vi "resonant.raw queue to image queue_MD.vi"() -> ()   [LabVIEW 2012]
uses:
  <vilib>/Utility/VariantDataType/Type.ctl
  GFG/GFGnumericGet.vi
  GFG/GFGbooleanGet.vi
  GFG/GFG library.lvlib
  <vilib>/Utility/VariantDataType/VariantType.lvlib
panel:
  out "size(s) 4":i32[](array[numeric])
  out "# elements in raw queue 2":i32
  out "error out 2":errorcluster
  out "error out 5":errorcluster
  out "size(s) 3":i32[](array[numeric])
  out "size(s) 2":i32[](array[numeric])
  out "size(s)":i32[](array[numeric])
  out "Numeric Control 2":i32
  out "Numeric Control":i32
  out "error out 4":errorcluster
  out "# elements in raw queue":i32
  out "error out":errorcluster
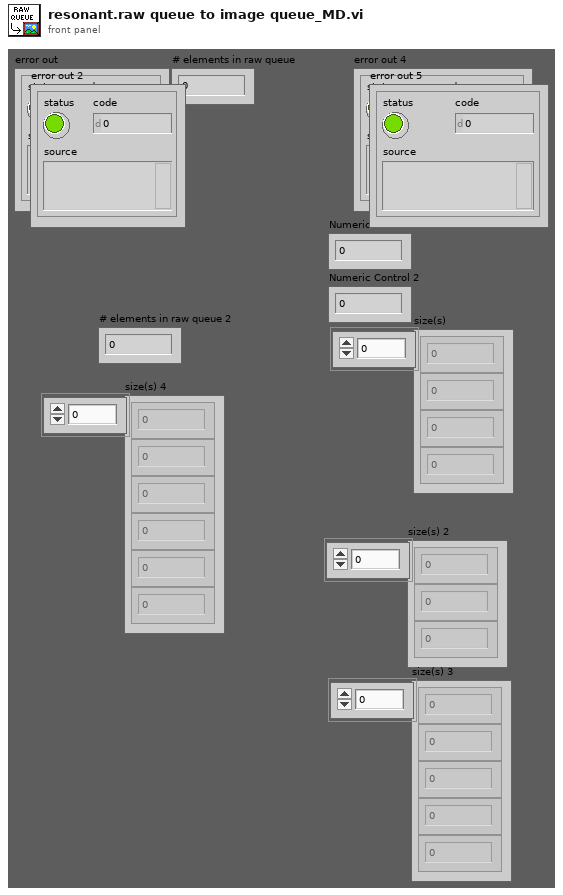
[diagram p1: front panel]
types:
  T1 = cluster{"NewVal":bool, "Event Registration Refnum":refnum<event-registration>}
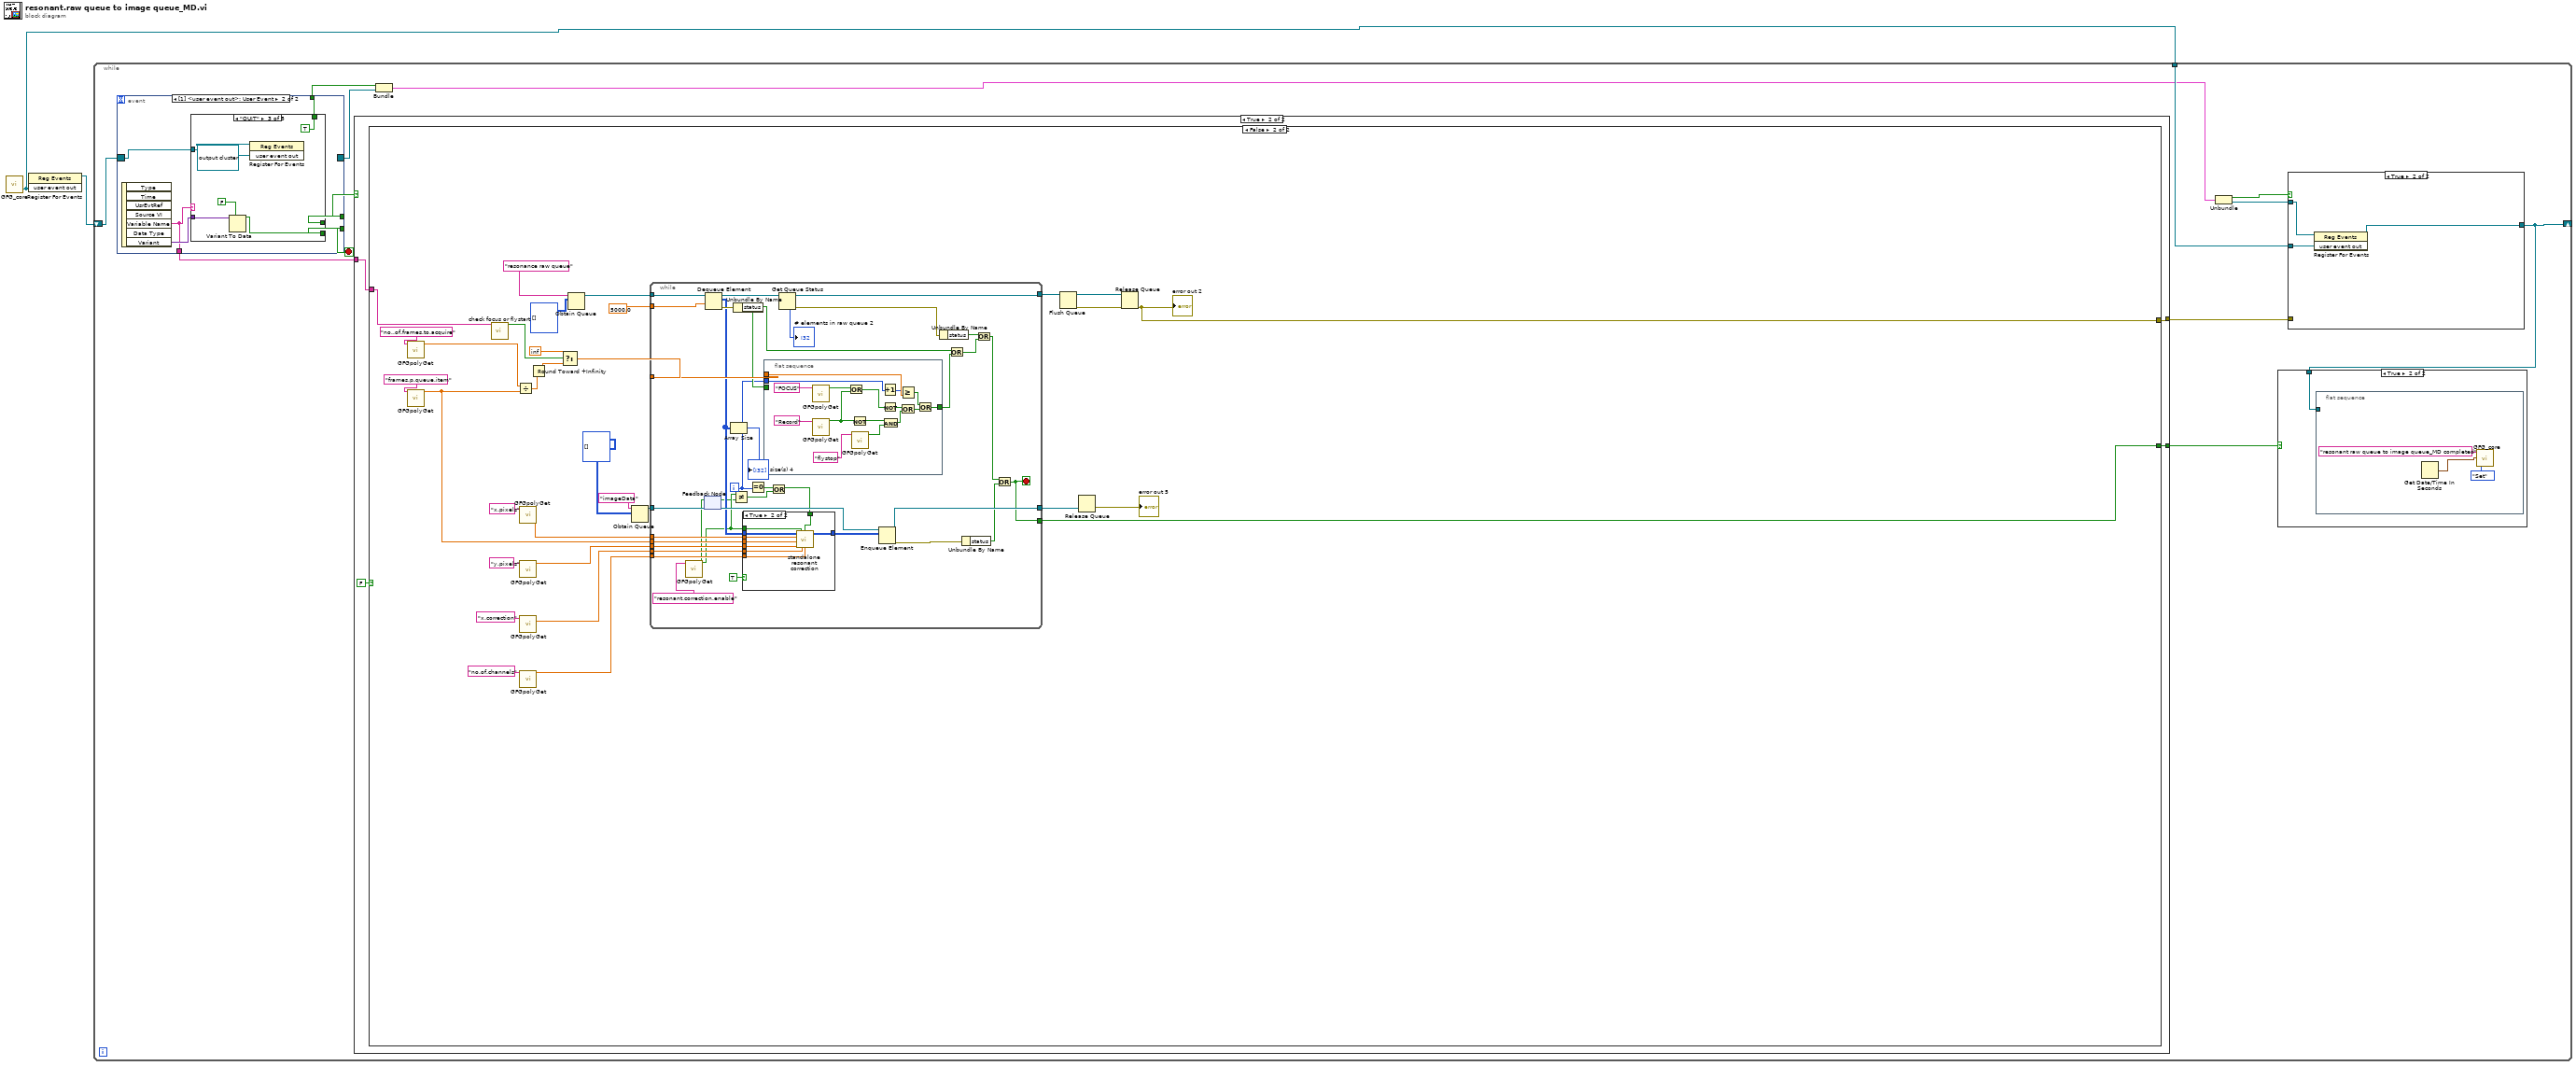
[diagram p0: block diagram]
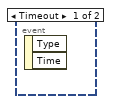
[diagram p4: hidden frame]
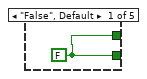
[diagram p5: hidden frame]
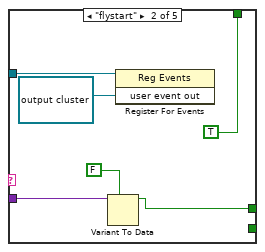
[diagram p6: hidden frame]
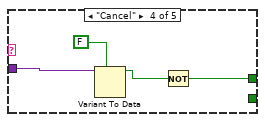
[diagram p7: hidden frame]
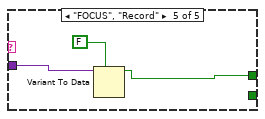
[diagram p8: hidden frame]
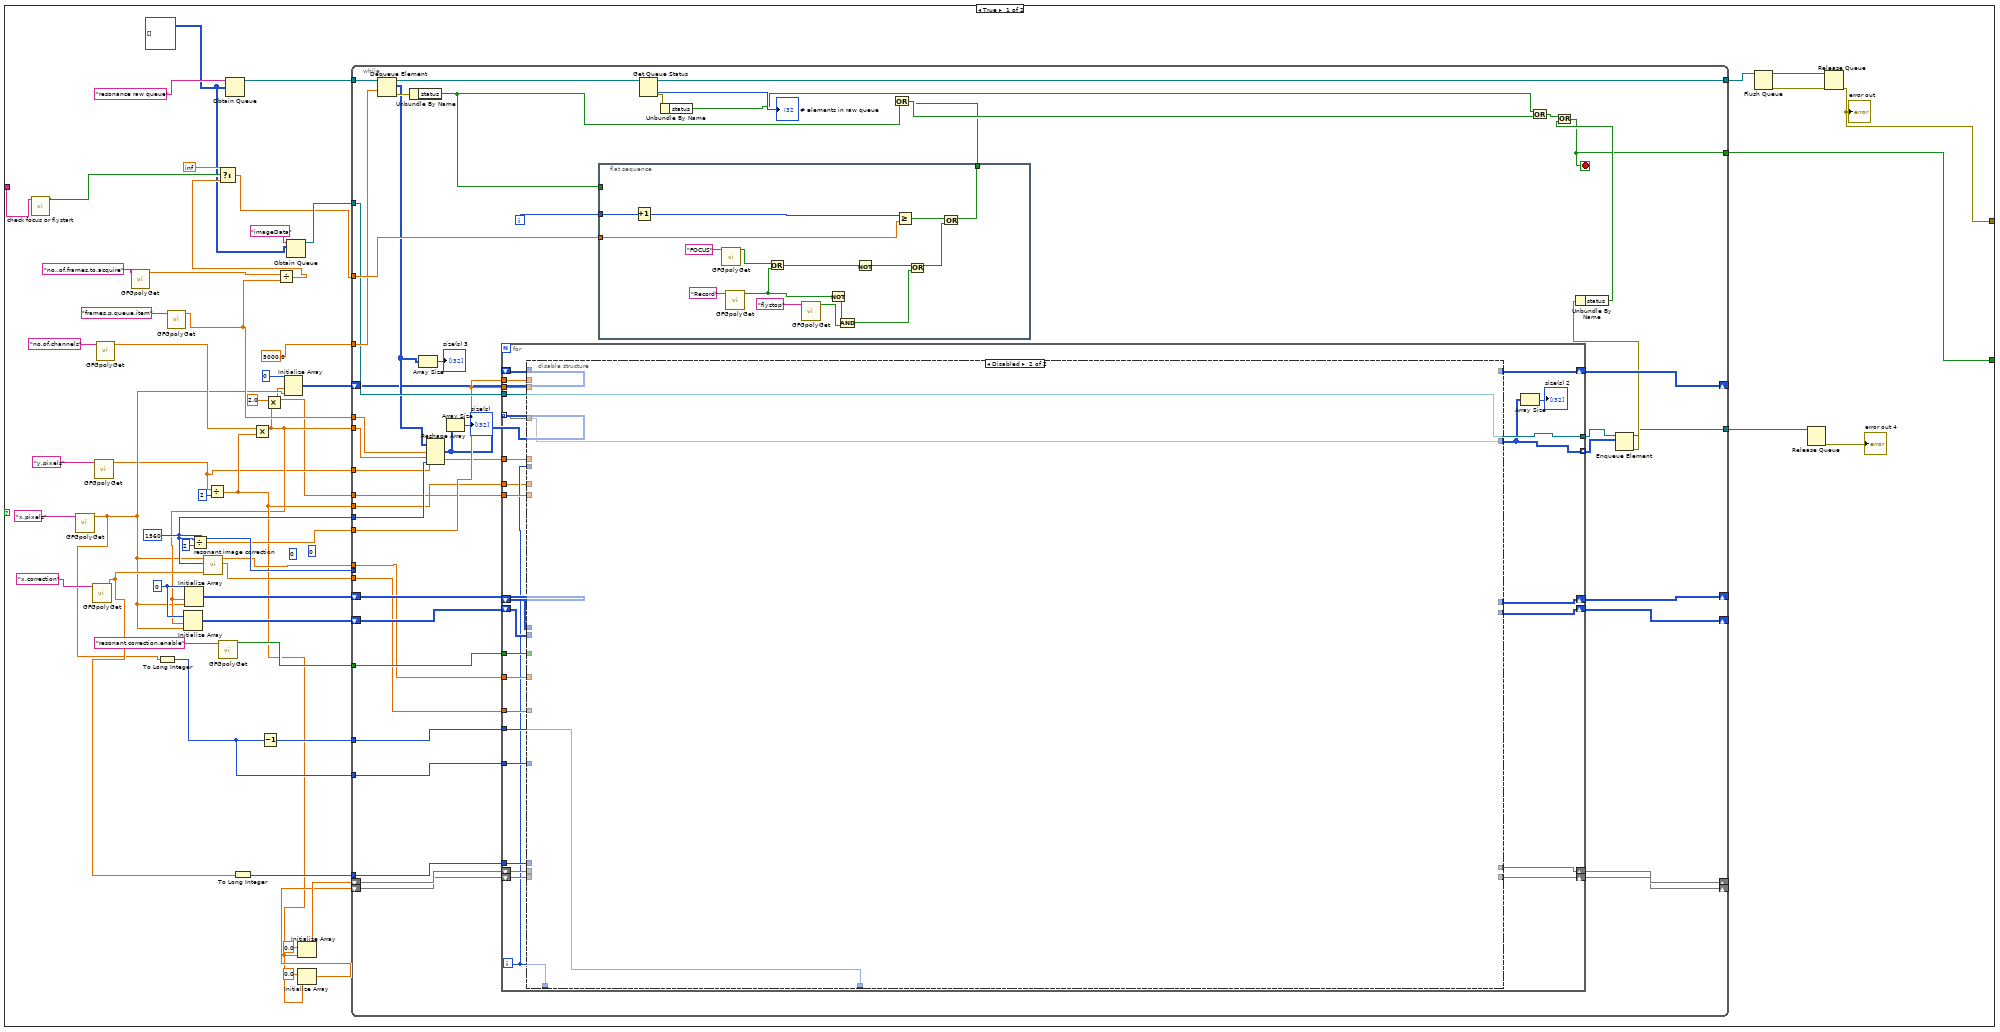
[diagram p10: hidden frame]
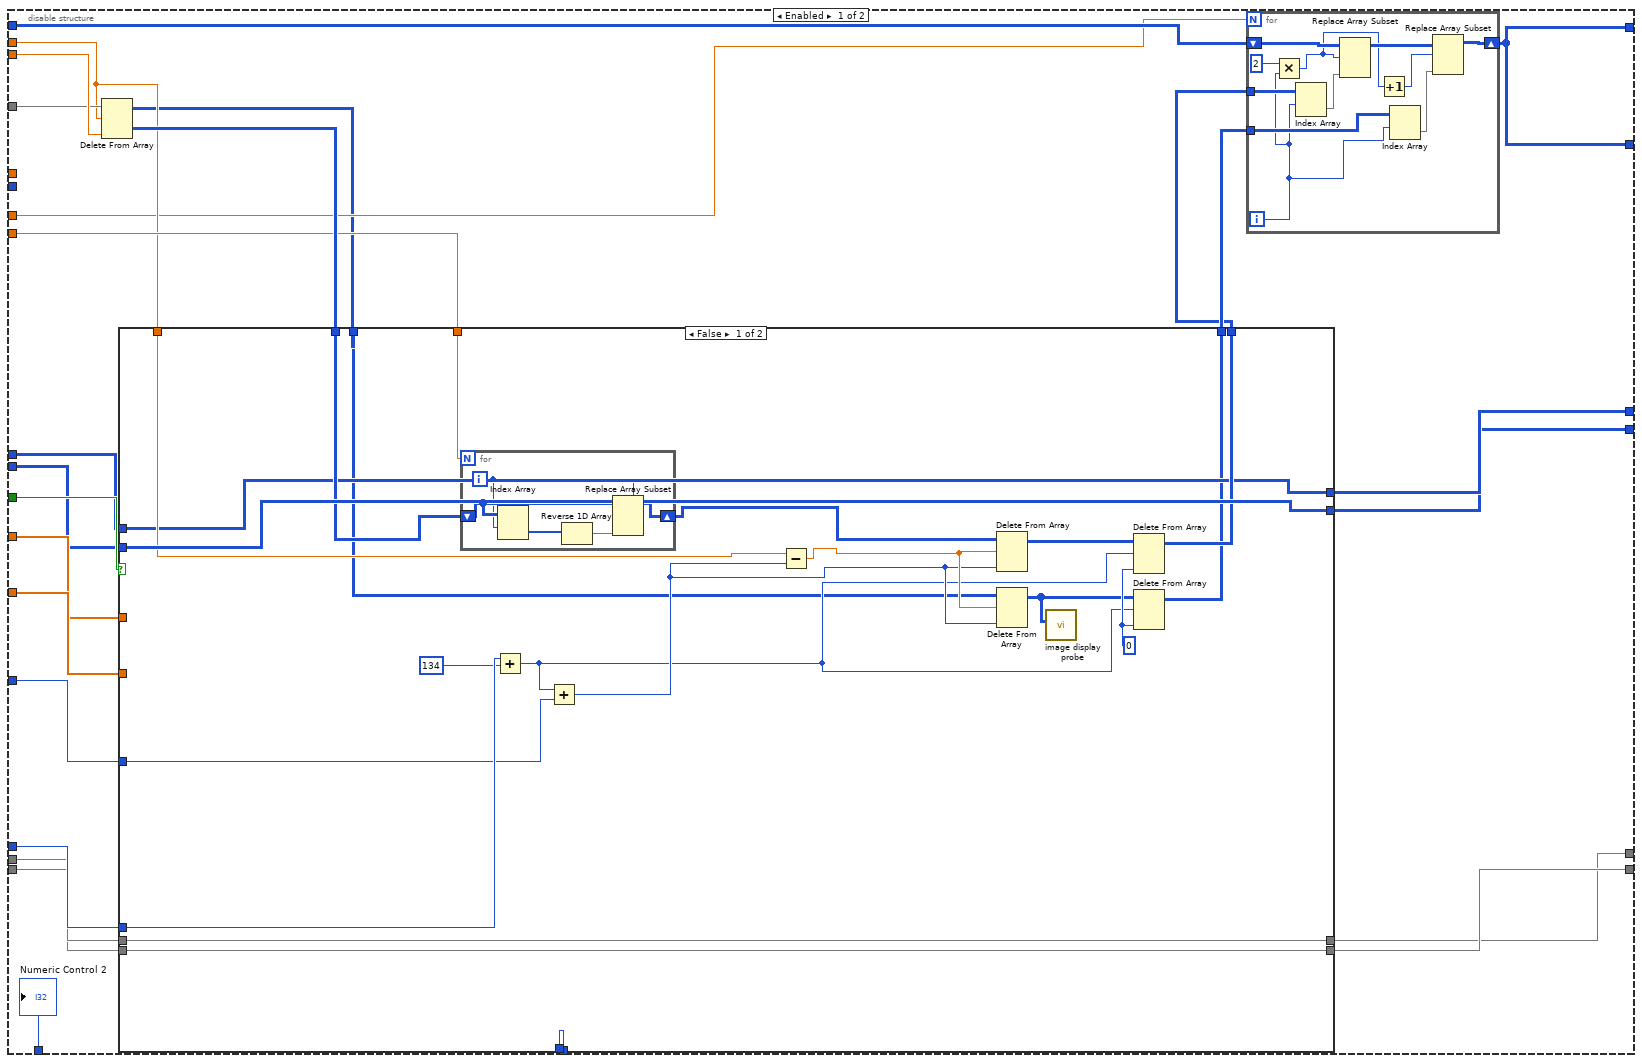
[diagram p11: hidden frame]
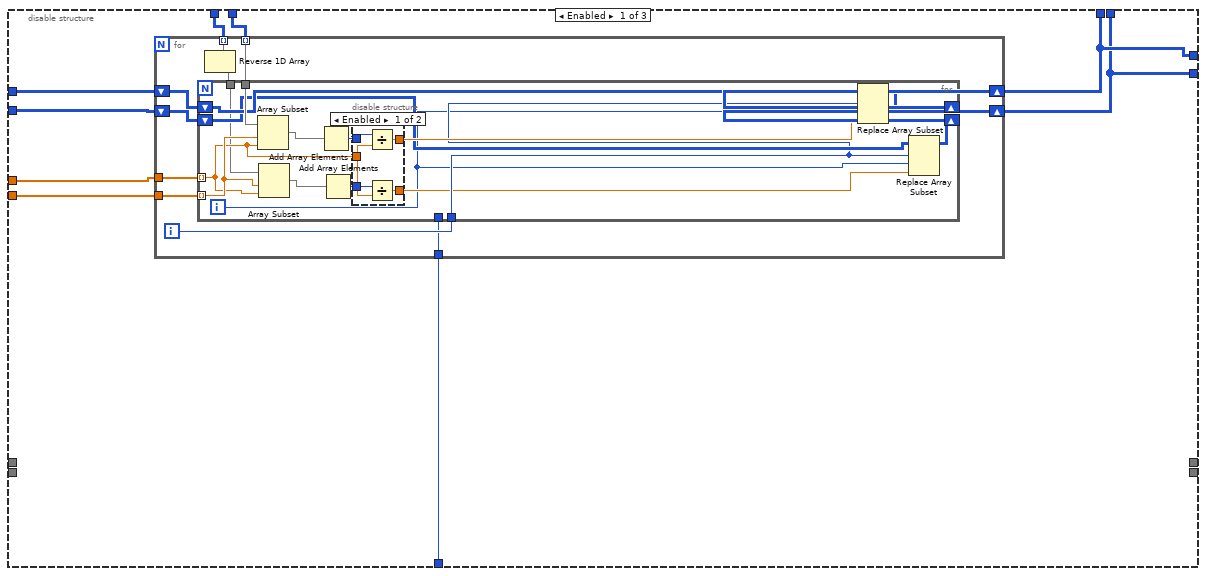
[diagram p13: hidden frame]
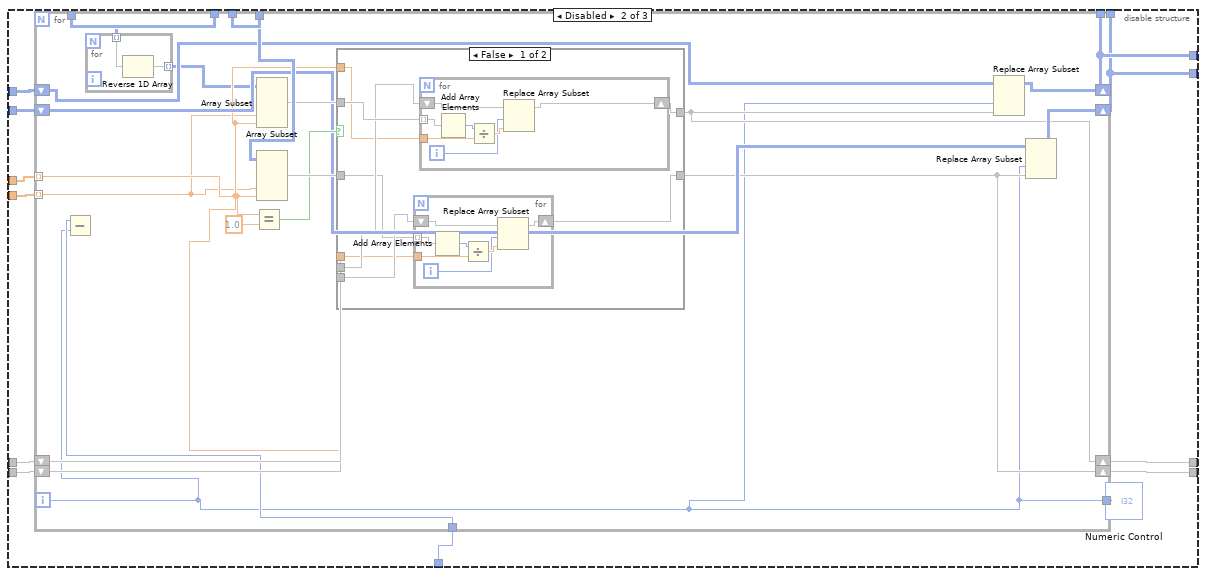
[diagram p15: hidden frame]
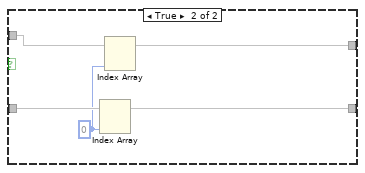
[diagram p16: hidden frame]
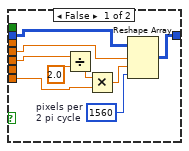
[diagram p17: hidden frame]
diagram:
  n1 = call "GFG_core.vi"() -> ("user event out"=w2:refnum<user-event>)  [unwired: 13 in, 6 out]
  n2 = register-events(w2) -> (reference out=w1:refnum<event-registration>)  [unwired: 2 in, 1 out]
  n3 = while {
    shift-right: [w3] -> _
    shift-left: w1 -> [w11]
    tunnel: w2 -> [w13]
    stop <- w14 stop-if-true
    n4 = event shown="[1] <user event out>: User Event" {
      selector: w11 -> [_ w26]
      dyn-events: [_ _] -> w9
      timeout: _ -> [_ _]
      tunnel: [_ w29] -> w15
      tunnel: [_ w28] -> w14
      tunnel: [_ w25] -> w10
      tunnel: [_ w24] -> w5
      event Timeout {
        n5 = event-data() -> ()  [unwired: 1 in, 2 out]
      }
      event User Event {
        n6 = event-data() -> ("Variable Name"=w24:string, "Variant"=w27:variant)  [unwired: 1 in, 5 out]
        n7 = case shown="\"QUIT\"" w24 {
          tunnel: [w30 w34 _ w43 w47] -> w29
          tunnel: [w30 _ w40 _ _] -> w28
          tunnel: w27 -> [_ w35 w42 w45 w48]
          tunnel: w26 -> [_ w32 w38 _ _]
          tunnel: [_ TRUE ("NewVal") TRUE ("NewVal") _ _] -> w25
          frame "False", Default {
            w30 = FALSE ("NewVal")
          }
          frame "flystart" {
            n8 = Variant To Data(type=FALSE ("NewVal"), Variant=w35) -> (data=w34:bool)  [unwired: 1 in, 1 out]
            n9 = register-events(reference=w32, refnum<user-event> refnum ("user event out")) -> ()  [unwired: 1 in, 2 out]
          }
          frame "QUIT" {
            n10 = Variant To Data(type=FALSE ("NewVal"), Variant=w42) -> (data=w40:bool)  [unwired: 1 in, 1 out]
            n11 = register-events(reference=w38, refnum<user-event> refnum ("user event out")) -> ()  [unwired: 1 in, 2 out]
          }
          frame "Cancel" {
            n12 = Variant To Data(type=FALSE ("NewVal"), Variant=w45) -> (data=w44:bool)  [unwired: 1 in, 1 out]
            n13 = Not(x=w44) -> (.not. x?=w43:bool)
          }
          frame "FOCUS", "Record" {
            n14 = Variant To Data(type=FALSE ("NewVal"), Variant=w48) -> (data=w47:bool)  [unwired: 1 in, 1 out]
          }
        }
      }
    }
    n15 = case shown="True" w15 {
      tunnel: [_ w53] -> w12
      tunnel: w5 -> [_ w52]
      tunnel: [_ w51] -> w4
      frame False {
      }
      frame True {
        n16 = case shown="False" FALSE {
          tunnel: [w75 w396] -> w53
          tunnel: w52 -> [w71 w393]
          tunnel: [w69 w391] -> w51
          frame True {
            (unwired) u32 0
            (unwired) u32 0
            w90 = i16 0 ("sum")
            w84 = 1560 ("dimension size")
            w54 = i16[][][] [] ("initialized array")
            n17 = call "check focus or flystart.vi"("x"=w71) -> ("x .or. y?"=w70:bool)  [unwired: 10 in]
            n18 = call-poly "GFGpolyGet.vi"("Variable Name in"="x.pixels" ("Tag in")) -> ("Numeric"=w58:dbl)  [unwired: 9 in, 1 out]
            n19 = call-poly "GFGpolyGet.vi"("Variable Name in"="x.correction" ("Tag in")) -> ("Numeric"=w85:dbl)  [unwired: 9 in, 1 out]
            n20 = call-poly "GFGpolyGet.vi"("Variable Name in"="y.pixels" ("Tag in")) -> ("Numeric"=w56:dbl)  [unwired: 9 in, 1 out]
            n21 = call-poly "GFGpolyGet.vi"("Variable Name in"="no.of.channels" ("Tag in")) -> ("Numeric"=w67:dbl)  [unwired: 9 in, 1 out]
            n22 = call-poly "GFGpolyGet.vi"("Variable Name in"="no..of.frames.to.acquire" ("Tag in")) -> ("Numeric"=w99:dbl)  [unwired: 9 in, 1 out]
            n23 = To Long Integer(number=w58) -> (32bit integer=w66:i32)
            n24 = call-poly "GFGpolyGet.vi"("Variable Name in"="frames.p.queue.item" ("Tag in")) -> ("Numeric"=w63:dbl)  [unwired: 9 in, 1 out]
            n25 = Divide(x=w84, y=2) -> (x/y=w83:dbl)
            n26 = call "resonant image correction.vi"("shift index"=w85, "pixels per period (2pi, 2 lines)"=w84, "x pixels"=w58) -> ("histogram cumsum"=w77:dbl[], "histogram pixels to avg"=w76:dbl[])  [unwired: 7 in]
            n27 = Divide(x=w56, y=2) -> (x/y=w62:dbl)
            n28 = call-poly "GFGpolyGet.vi"("Variable Name in"="resonant.correction.enable" ("Tag in")) -> ("Boolean"=w92:bool)  [unwired: 10 in]
            n29 = Obtain Queue(name (unnamed)="resonance raw queue", element data type=w54) -> (queue out=w104:refnum<queue>)  [unwired: 3 in, 2 out]
            n30 = To Long Integer(number=w85) -> (32bit integer=w65:i32)
            n31 = Multiply(x=w67, y=w62) -> (x*y=w60:dbl)
            n32 = Initialize Array(w90, w60, w58) -> (w89:i16[][])
            n33 = Initialize Array(w90, w60, w58) -> (w88:i16[][])
            n34 = Decrement(x=w66) -> (x-1=w87:i32)
            n35 = Multiply(x=2.0, y=w60) -> (x*y=w55:dbl)
            n36 = Divide(x=w99, y=w63) -> (x/y=w73:dbl)
            n37 = Select(t=inf, s=w70, f=w73) -> (s? t:f=w72:dbl)
            n38 = Initialize Array(i16 0 ("sum"), w55, w58) -> (w57:i16[][])
            n39 = Obtain Queue(name (unnamed)="imageData", element data type=w54) -> (queue out=w105:refnum<queue>)  [unwired: 3 in, 2 out]
            n40 = Initialize Array(0.0 ("element"), w62) -> (w80:dbl[])
            n41 = Initialize Array(0.0 ("element"), w62) -> (w78:dbl[])
            n42 = while {
              tunnel: w104 -> [w150]
              tunnel: [w147] -> w103
              tunnel: w105 -> [w145]
              tunnel: w72 -> [w154]
              tunnel: 5000.0 -> [w151]
              tunnel: [w108] -> w96
              tunnel: w84 -> [w144]
              tunnel: w83 -> [w143]
              tunnel: w92 -> [w142]
              tunnel: w87 -> [w139]
              tunnel: w84 -> [_]
              tunnel: w77 -> [w134]
              tunnel: w76 -> [w133]
              tunnel: w65 -> [w132]
              shift-right: [w129] -> _
              shift-left: w80 -> [w131]
              shift-right: [w128] -> _
              shift-left: w78 -> [w130]
              shift-right: [w126] -> _
              shift-left: w89 -> [w141]
              shift-right: [w127] -> _
              shift-left: w88 -> [w140]
              tunnel: w66 -> [w125]
              tunnel: [w124] -> w69
              tunnel: w60 -> [w118]
              tunnel: w63 -> [w119]
              tunnel: w62 -> [w117]
              shift-right: [w115] -> _
              shift-left: w57 -> [w116]
              tunnel: w56 -> [w114]
              tunnel: w55 -> [w113]
              i -> [w152]
              stop <- w124 stop-if-true
              n43 = Dequeue Element(queue=w150, timeout in ms (-1)=w151) -> (queue out=w148:refnum<queue>, element=w121:i16[][][], error out=w153:errorcluster)  [unwired: 1 in, 1 out]
              n44 = Unbundle By Name(w153) -> ("status"=w123:bool)
              n45 = Array Size(array=w121) -> (size(s)=→"size(s) 3":i32[])
              n46 = Reshape Array(w121, w119, w118, w144) -> (w112:i16[][][])
              n47 = Array Size(array=w112) -> (size(s)=→"size(s)":i32[])
              n48 = for {
                tunnel: w112 -> [w181] mode=indexing
                tunnel: w143 -> [w197]
                tunnel: w143 -> [w196]
                tunnel: w145 -> [w173]
                tunnel: [w173] -> w110
                tunnel: w142 -> [w195]
                tunnel: w134 -> [w194]
                tunnel: w133 -> [w193]
                tunnel: w139 -> [w190]
                tunnel: [w172] -> w109 mode=indexing
                tunnel: w132 -> [w189]
                shift-right: [w185] -> w129
                shift-left: w131 -> [w188]
                shift-right: [w186] -> w128
                shift-left: w130 -> [w187]
                shift-right: [w184] -> w127
                shift-left: w140 -> [w191]
                shift-right: [w183] -> w126
                shift-left: w141 -> [w192]
                tunnel: w125 -> [w182]
                tunnel: w117 -> [w179]
                shift-right: [w177] -> w115
                shift-left: w116 -> [w178]
                tunnel: w114 -> [w175]
                tunnel: w113 -> [w174]
                i -> [w176]
                n49 = disable-structure shown="Disabled" {
                  disable-tunnel: w197 -> [w202 _]
                  disable-tunnel: w196 -> [w223 _]
                  disable-tunnel: w195 -> [w222 _]
                  disable-tunnel: w194 -> [w221 _]
                  disable-tunnel: w193 -> [w220 _]
                  disable-tunnel: w192 -> [w219 _]
                  disable-tunnel: w191 -> [w218 _]
                  disable-tunnel: [w200 w380] -> w172
                  disable-tunnel: w190 -> [w216 _]
                  disable-tunnel: w189 -> [w215 _]
                  disable-tunnel: w188 -> [w214 _]
                  disable-tunnel: w187 -> [w213 _]
                  disable-tunnel: [w212 _] -> w186
                  disable-tunnel: [w211 _] -> w185
                  disable-tunnel: [w210 _] -> w184
                  disable-tunnel: [w209 _] -> w183
                  disable-tunnel: w182 -> [w208 _]
                  disable-tunnel: w176 -> [w207 _]
                  disable-tunnel: w181 -> [w205 w380]
                  disable-tunnel: w179 -> [w206 _]
                  disable-tunnel: w178 -> [w203 _]
                  disable-tunnel: [w200 _] -> w177
                  disable-tunnel: w176 -> [_ _]
                  disable-tunnel: w175 -> [_ _]
                  disable-tunnel: w174 -> [w201 _]
                  frame Enabled {
                    n50 = Delete From Array(array=w205, length=w202, index (col)=w223) -> (deleted portion=w217:i16[][], array with subset deleted=w198:i16[][])  [unwired: 1 in]
                    n51 = case shown="False" w222 {
                      tunnel: w217 -> [w230 w263]
                      tunnel: w198 -> [w226 w262]
                      tunnel: w221 -> [_ w261]
                      tunnel: w220 -> [_ w260]
                      tunnel: w219 -> [w239 w259]
                      tunnel: w218 -> [w228 w258]
                      tunnel: [w225 w257] -> w204
                      tunnel: [w237 w256] -> w199
                      tunnel: w216 -> [_ w255]
                      tunnel: w215 -> [w242 _]
                      tunnel: w214 -> [w241 w254]
                      tunnel: [w241 w253] -> w211
                      tunnel: w213 -> [w240 w252]
                      tunnel: [w240 w251] -> w212
                      tunnel: [w228 w250] -> w210
                      tunnel: [w239 w249] -> w209
                      tunnel: w208 -> [w236 _]
                      tunnel: w206 -> [w231 _]
                      tunnel: w202 -> [w229 _]
                      frame False {
                        w243 = 0 ("disabled index (col)")
                        n52 = for {
                          N: w231 -> [_]
                          shift-right: [w247] -> w227
                          shift-left: w230 -> [w246]
                          i -> [w245]
                          n53 = Index Array(array=w246, index (row)=w245) -> (element=w244:i16[])  [unwired: 1 in]
                          n54 = Reverse 1D Array(array=w244) -> (reversed array=w248:i16[])
                          n55 = Replace Array Subset(array=w246, new element=w248, index (row)=w245) -> (w247:i16[][])  [unwired: 1 in]
                        }
                        n56 = Add(x=w242, y=134 ("length")) -> (x+y=w232:i32)
                        n57 = Add(x=w232, y=w236) -> (x+y=w233:i32)
                        n58 = Subtract(x=w229, y=w233) -> (x-y=w234:dbl)
                        n59 = Delete From Array(array=w227, length=w234, index (col)=w233) -> (array with subset deleted=w238:i16[][])  [unwired: 1 in, 1 out]
                        n60 = Delete From Array(array=w226, length=w234, index (col)=w233) -> (array with subset deleted=w224:i16[][])  [unwired: 1 in, 1 out]
                        n61 = call "image display probe.vi"("Image Pixels (I16)"=w224) -> ()  [unwired: 11 in]
                        n62 = Delete From Array(array=w238, length=w232, index (col)=w243) -> (array with subset deleted=w237:i16[][])  [unwired: 1 in, 1 out]
                        n63 = Delete From Array(array=w224, length=w232, index (col)=w243) -> (array with subset deleted=w225:i16[][])  [unwired: 1 in, 1 out]
                      }
                      frame True {
                        n64 = disable-structure shown="Disabled" {
                          disable-tunnel: w263 -> [w272 w320 _]
                          disable-tunnel: w262 -> [w271 w319 _]
                          disable-tunnel: w261 -> [w270 w318 _]
                          disable-tunnel: w260 -> [w269 w307 _]
                          disable-tunnel: w259 -> [w268 w317 _]
                          disable-tunnel: w258 -> [w267 w316 _]
                          disable-tunnel: [w265 w310 _] -> w257
                          disable-tunnel: [w264 w309 _] -> w256
                          disable-tunnel: w255 -> [w266 w315 _]
                          disable-tunnel: w254 -> [_ w314 _]
                          disable-tunnel: [_ w313 _] -> w253
                          disable-tunnel: w252 -> [_ w312 _]
                          disable-tunnel: [_ w311 _] -> w251
                          disable-tunnel: [w265 w310 _] -> w250
                          disable-tunnel: [w264 w309 _] -> w249
                          frame Enabled {
                            n65 = for {
                              tunnel: w272 -> [w281] mode=indexing
                              tunnel: w271 -> [w280] mode=indexing
                              tunnel: w270 -> [w283]
                              tunnel: w269 -> [w282]
                              shift-right: [w275] -> w264
                              shift-left: w268 -> [w279]
                              shift-right: [w276] -> w265
                              shift-left: w267 -> [w278]
                              tunnel: w266 -> [w274]
                              i -> [w277]
                              n66 = Reverse 1D Array(array=w281) -> (reversed array=w273:i16[])
                              n67 = for {
                                tunnel: w283 -> [w298] mode=indexing
                                tunnel: w282 -> [w293] mode=indexing
                                tunnel: w273 -> [w284]
                                tunnel: w280 -> [w299]
                                shift-right: [w286] -> w275
                                shift-left: w279 -> [w290]
                                shift-right: [w287] -> w276
                                shift-left: w278 -> [w291]
                                tunnel: w277 -> [w289]
                                tunnel: w274 -> [_]
                                i -> [w285]
                                n68 = Array Subset(array=w299, index=w298, length=w293) -> (w297:i16[])
                                n69 = Array Subset(array=w284, index=w298, length=w293) -> (w296:i16[])
                                n70 = Add Array Elements(numeric array=w297) -> (sum=w295:i16)
                                n71 = Add Array Elements(numeric array=w296) -> (sum=w294:i16)
                                n72 = disable-structure shown="Enabled" {
                                disable-tunnel: w295 -> [w304 w306]
                                disable-tunnel: w294 -> [w303 w305]
                                disable-tunnel: w293 -> [w302 _]
                                disable-tunnel: [w301 w306] -> w292
                                disable-tunnel: [w300 w305] -> w288
                                frame Enabled {
                                n73 = Divide(x=w304, y=w302) -> (x/y=w301:dbl)
                                n74 = Divide(x=w303, y=w302) -> (x/y=w300:dbl)
                                }
                                frame Disabled {
                                }
                                }
                                n75 = Replace Array Subset(array=w291, new element=w292, index (row)=w289, index (col)=w285) -> (w287:i16[][])
                                n76 = Replace Array Subset(array=w290, new element=w288, index (row)=w289, index (col)=w285) -> (w286:i16[][])
                              }
                            }
                          }
                          frame Disabled {
                            n77 = for {
                              tunnel: w320 -> [w322]
                              tunnel: w319 -> [w339]
                              tunnel: w318 -> [w323] mode=indexing
                              tunnel: w307 -> [w324] mode=indexing
                              shift-right: [w333] -> w309
                              shift-left: w317 -> [w332]
                              shift-right: [w334] -> w310
                              shift-left: w316 -> [w331]
                              tunnel: w315 -> [w326]
                              shift-right: [w328] -> w313
                              shift-left: w314 -> [w330]
                              shift-right: [w327] -> w311
                              shift-left: w312 -> [w329]
                              tunnel: [w325] -> w308
                              i -> [w325]
                              n78 = Subtract(x=w326, y=w325) -> ()  [unwired: 1 out]
                              n79 = for {
                                tunnel: w322 -> [w341] mode=indexing
                                tunnel: [w340] -> w321 mode=indexing
                                n80 = Reverse 1D Array(array=w341) -> (reversed array=w340:i16[])
                              }
                              n81 = Equal?(x=w324, y=1.0) -> (x = y?=w335:bool)
                              n82 = Array Subset(array=w321, index (col)=w323, length (col)=w324) -> (w337:i16[][])  [unwired: 2 in]
                              n83 = Array Subset(array=w339, index (col)=w323, length (col)=w324) -> (w338:i16[][])  [unwired: 2 in]
                              n84 = case shown="False" w335 {
                                tunnel: w338 -> [w345 w367]
                                tunnel: w337 -> [w349 w368]
                                tunnel: [w347 w366] -> w328
                                tunnel: [w343 w365] -> w327
                                tunnel: w324 -> [w344 _]
                                tunnel: w330 -> [w348 _]
                                tunnel: w329 -> [w346 _]
                                tunnel: w324 -> [w342 _]
                                frame False {
                                n85 = for {
                                tunnel: w345 -> [w356] mode=indexing
                                shift-right: [w350] -> w343
                                shift-left: w346 -> [w353]
                                tunnel: w342 -> [w354]
                                i -> [w351]
                                n86 = Add Array Elements(numeric array=w356) -> (sum=w355:i16)
                                n87 = Divide(x=w355, y=w354) -> (x/y=w352:dbl)
                                n88 = Replace Array Subset(array=w353, new element=w352, index=w351) -> (w350:dbl[])
                                }
                                n89 = for {
                                tunnel: w349 -> [w363] mode=indexing
                                shift-right: [w358] -> w347
                                shift-left: w348 -> [w360]
                                tunnel: w344 -> [w361]
                                i -> [w357]
                                n90 = Add Array Elements(numeric array=w363) -> (sum=w362:i16)
                                n91 = Divide(x=w362, y=w361) -> (x/y=w359:dbl)
                                n92 = Replace Array Subset(array=w360, new element=w359, index=w357) -> (w358:dbl[])
                                }
                                }
                                frame True {
                                w364 = 0 ("disabled index (col)")
                                n93 = Index Array(array=w367, index (col)=w364) -> (element=w365:i16[])  [unwired: 1 in]
                                n94 = Index Array(array=w368, index (col)=w364) -> (element=w366:i16[])  [unwired: 1 in]
                                }
                              }
                              n95 = Replace Array Subset(array=w331, new element=w328, index (col)=w325) -> (w334:i16[][])  [unwired: 1 in]
                              n96 = Replace Array Subset(array=w332, new element=w327, index (col)=w325) -> (w333:i16[][])  [unwired: 1 in]
                            }
                            "Numeric Control" <- w308
                          }
                          frame Disabled {
                          }
                        }
                      }
                    }
                    n97 = for {
                      N: w201 -> [_]
                      shift-right: [w375] -> w200
                      shift-left: w203 -> [w377]
                      tunnel: w199 -> [w379]
                      tunnel: w204 -> [w378]
                      i -> [w370]
                      n98 = Multiply(x=2, y=w370) -> (x*y=w369:i32)
                      n99 = Index Array(array=w379, index (row)=w370) -> (element=w374:i16[])  [unwired: 1 in]
                      n100 = Replace Array Subset(array=w377, new element=w374, index (row)=w369) -> (w376:i16[][])  [unwired: 1 in]
                      n101 = Increment(x=w369) -> (x+1=w371:i32)
                      n102 = Index Array(array=w378, index (row)=w370) -> (element=w373:i16[])  [unwired: 1 in]
                      n103 = Replace Array Subset(array=w376, new element=w373, index (row)=w371) -> (w375:i16[][])  [unwired: 1 in]
                    }
                    "Numeric Control 2" <- w207
                  }
                  frame Disabled {
                  }
                }
                n104 = Array Size(array=w172) -> (size(s)=→"size(s) 2":i32[])
              }
              n105 = flat-sequence {
                tunnel: w154 -> [w171]
                tunnel: w152 -> [w169]
                tunnel: [w165] -> w149
                tunnel: w123 -> [_]
                frame #0 {
                  n106 = Increment(x=w169) -> (x+1=w163:i32)
                  n107 = call-poly "GFGpolyGet.vi"("Variable Name in"="FOCUS") -> ("Boolean"=w166:bool)  [unwired: 10 in]
                  n108 = call-poly "GFGpolyGet.vi"("Variable Name in"="Record") -> ("Boolean"=w158:bool)  [unwired: 10 in]
                  n109 = Or(x=w166, y=w158) -> (x .or. y?=w164:bool)
                  n110 = call-poly "GFGpolyGet.vi"("Variable Name in"="flystop") -> ("Boolean"=w159:bool)  [unwired: 10 in]
                  n111 = Not(x=w158) -> (.not. x?=w160:bool)
                  n112 = And(x=w160, y=w159) -> (x .and. y?=w156:bool)
                  n113 = Not(x=w164) -> (.not. x?=w162:bool)
                  n114 = Greater Or Equal?(x=w163, y=w171) -> (x >= y?=w170:bool)
                  n115 = Or(x=w162, y=w156) -> (x .or. y?=w157:bool)
                  n116 = Or(x=w170, y=w157) -> (x .or. y?=w165:bool)
                }
              }
              n117 = Get Queue Status(queue=w148) -> (queue out=w147:refnum<queue>, error out=w137:errorcluster, # elements in queue=→"# elements in raw queue":i32)  [unwired: 2 in, 5 out]
              n118 = Unbundle By Name(w137) -> ("status"=w136:bool)
              n119 = Or(x=w123, y=w149) -> (x .or. y?=w155:bool)
              n120 = Or(x=w136, y=w155) -> (x .or. y?=w138:bool)
              n121 = Enqueue Element(queue=w110, element=w109) -> (queue out=w108:refnum<queue>, error out=w111:errorcluster)  [unwired: 2 in, 1 out]
              n122 = Unbundle By Name(w111) -> ("status"=w135:bool)
              n123 = Or(x=w138, y=w135) -> (x .or. y?=w124:bool)
            }
            n124 = Flush Queue(queue=w103) -> (queue out=w102:refnum<queue>, error out=w98:errorcluster)  [unwired: 1 in, 1 out]
            n125 = Release Queue(queue=w96) -> (error out=→"error out 4":errorcluster)  [unwired: 2 in, 2 out]
            n126 = Release Queue(queue=w102, error in (no error)=w98) -> (error out=w75:errorcluster)  [unwired: 1 in, 2 out]
            "error out" <- w75
          }
          frame False {
            n127 = call-poly "GFGpolyGet.vi"("Variable Name in"="no..of.frames.to.acquire" ("Tag in")) -> ("Numeric"=w404:dbl)  [unwired: 9 in, 1 out]
            n128 = call-poly "GFGpolyGet.vi"("Variable Name in"="frames.p.queue.item" ("Tag in")) -> ("Numeric"=w387:dbl)  [unwired: 9 in, 1 out]
            n129 = call "check focus or flystart.vi"("x"=w393) -> ("x .or. y?"=w392:bool)  [unwired: 10 in]
            n130 = Divide(x=w404, y=w387) -> (x/y=w381:dbl)
            n131 = call-poly "GFGpolyGet.vi"("Variable Name in"="x.pixels" ("Tag in")) -> ("Numeric"=w386:dbl)  [unwired: 9 in, 1 out]
            n132 = call-poly "GFGpolyGet.vi"("Variable Name in"="y.pixels" ("Tag in")) -> ("Numeric"=w388:dbl)  [unwired: 9 in, 1 out]
            n133 = call-poly "GFGpolyGet.vi"("Variable Name in"="x.correction" ("Tag in")) -> ("Numeric"=w385:dbl)  [unwired: 9 in, 1 out]
            n134 = call-poly "GFGpolyGet.vi"("Variable Name in"="no.of.channels" ("Tag in")) -> ("Numeric"=w384:dbl)  [unwired: 9 in, 1 out]
            n135 = Round Toward +Infinity(x=w381) -> (ceil(x): smallest int >= x=w382:dbl)
            n136 = Select(t=inf, s=w392, f=w382) -> (s? t:f=w394:dbl)
            n137 = Obtain Queue(name (unnamed)="resonance raw queue", element data type=i16[][][] [] ("initialized array")) -> (queue out=w409:refnum<queue>)  [unwired: 3 in, 2 out]
            n138 = Obtain Queue(name (unnamed)="imageData", element data type=i16[][][] [] ("initialized array")) -> (queue out=w410:refnum<queue>)  [unwired: 3 in, 2 out]
            n139 = while {
              tunnel: w409 -> [w442]
              tunnel: [w439] -> w408
              tunnel: w410 -> [w437]
              tunnel: w394 -> [w445]
              tunnel: 5000.0 -> [w443]
              tunnel: [w436] -> w400
              tunnel: [w430] -> w391
              tunnel: w388 -> [w426]
              tunnel: w387 -> [w425]
              tunnel: w386 -> [w424]
              tunnel: w385 -> [w423]
              tunnel: w384 -> [w422]
              i -> [w428]
              stop <- w430 stop-if-true
              n140 = call-poly "GFGpolyGet.vi"("Variable Name in"="resonant.correction.enable" ("Tag in")) -> ("Boolean"=w415:bool)  [unwired: 10 in]
              n141 = feedback-in #1(w415) -> ()
              n142 = feedback #1() -> (w414:bool)  [unwired: 1 in]
              n143 = Dequeue Element(queue=w442, timeout in ms (-1)=w443) -> (queue out=w440:refnum<queue>, element=w420:i16[][][], error out=w444:errorcluster)  [unwired: 1 in, 1 out]
              n144 = Array Size(array=w420) -> (size(s)=→"size(s) 4":i32[])
              n145 = Not Equal?(x=w415, y=w414) -> (x != y?=w413:bool)
              n146 = Unbundle By Name(w444) -> ("status"=w429:bool)
              n147 = Equal To 0?(x=w428) -> (x = 0?=w427:bool)
              n148 = flat-sequence {
                tunnel: w445 -> [w480]
                tunnel: w428 -> [w478]
                tunnel: [w474] -> w441
                tunnel: w429 -> [_]
                frame #0 {
                  n149 = call-poly "GFGpolyGet.vi"("Variable Name in"="FOCUS") -> ("Boolean"=w475:bool)  [unwired: 10 in]
                  n150 = call-poly "GFGpolyGet.vi"("Variable Name in"="Record") -> ("Boolean"=w467:bool)  [unwired: 10 in]
                  n151 = Or(x=w475, y=w467) -> (x .or. y?=w473:bool)
                  n152 = Not(x=w467) -> (.not. x?=w469:bool)
                  n153 = call-poly "GFGpolyGet.vi"("Variable Name in"="flystop") -> ("Boolean"=w468:bool)  [unwired: 10 in]
                  n154 = Increment(x=w478) -> (x+1=w472:i32)
                  n155 = Not(x=w473) -> (.not. x?=w471:bool)
                  n156 = And(x=w469, y=w468) -> (x .and. y?=w465:bool)
                  n157 = Greater Or Equal?(x=w472, y=w480) -> (x >= y?=w479:bool)
                  n158 = Or(x=w471, y=w465) -> (x .or. y?=w466:bool)
                  n159 = Or(x=w479, y=w466) -> (x .or. y?=w474:bool)
                }
              }
              n160 = Or(x=w427, y=w413) -> (x .or. y?=w416:bool)
              n161 = case shown="True" TRUE {
                tunnel: w416 -> [_ w464]
                tunnel: w415 -> [_ w463]
                tunnel: w426 -> [w450 w462]
                tunnel: w425 -> [w448 w461]
                tunnel: w424 -> [_ w460]
                tunnel: w423 -> [_ w459]
                tunnel: w422 -> [w449 w458]
                tunnel: [w447 w457] -> w421
                tunnel: w420 -> [w451 w456]
                frame False {
                  w455 = 1560  # pixels per 2 pi cycle
                  n162 = Divide(x=w450, y=2.0) -> (x/y=w453:dbl)
                  n163 = Multiply(x=w453, y=w449) -> (x*y=w452:dbl)
                  n164 = Reshape Array(w451, w448, w452, w455) -> (w447:i16[][][])
                }
                frame True {
                  n165 = call "standalone resonant correction.vi"("uncorrected images in"=w456, "resonant.correction.enable"=w463, "force reset shift registers"=w464, "frames.p.queue.item"=w461, "x.pixels"=w460, "y.pixels"=w462, "x.correction"=w459, "no.of.channels"=w458) -> ("corrected images out"=w457:i16[][][])  [unwired: 7 in]
                }
              }
              n166 = Get Queue Status(queue=w440) -> (queue out=w439:refnum<queue>, error out=w434:errorcluster, # elements in queue=→"# elements in raw queue 2":i32)  [unwired: 2 in, 5 out]
              n167 = Enqueue Element(queue=w437, element=w421) -> (queue out=w436:refnum<queue>, error out=w432:errorcluster)  [unwired: 2 in, 1 out]
              n168 = Unbundle By Name(w434) -> ("status"=w433:bool)
              n169 = Or(x=w429, y=w441) -> (x .or. y?=w446:bool)
              n170 = Unbundle By Name(w432) -> ("status"=w431:bool)
              n171 = Or(x=w433, y=w446) -> (x .or. y?=w435:bool)
              n172 = Or(x=w435, y=w431) -> (x .or. y?=w430:bool)
            }
            n173 = Flush Queue(queue=w408) -> (queue out=w407:refnum<queue>, error out=w403:errorcluster)  [unwired: 1 in, 1 out]
            n174 = Release Queue(queue=w400) -> (error out=→"error out 5":errorcluster)  [unwired: 2 in, 2 out]
            n175 = Release Queue(queue=w407, error in (no error)=w403) -> (error out=w396:errorcluster)  [unwired: 1 in, 2 out]
            "error out 2" <- w396
          }
        }
      }
    }
    n176 = Bundle("NewVal"=w10, "Event Registration Refnum"=w9) -> (w8:T1)  [unwired: 1 in]
    n177 = Unbundle(w8) -> ("NewVal"=w7:bool, "Event Registration Refnum"=w6:refnum<event-registration>)
    n178 = case shown="True" w7 {
      tunnel: [w20 w23] -> w3
      tunnel: w13 -> [_ w22]
      tunnel: w12 -> [_ _]
      tunnel: w6 -> [w20 w21]
      frame False {
      }
      frame True {
        n179 = register-events(reference=w21, w22) -> (reference out=w23:refnum<event-registration>)  [unwired: 1 in, 1 out]
      }
    }
    n180 = case shown="True" w4 {
      tunnel: w3 -> [_ w16]
      frame False {
      }
      frame True {
        n181 = flat-sequence {
          tunnel: w16 -> [_]
          frame #0 {
            n182 = Get Date/Time In Seconds() -> (seconds since 1Jan1904=w17:timestamp)
            n183 = call "GFG_core.vi"("Variable Name in"="resonant raw queue to image queue_MD completed", "Variant in"=w17, "Action"=enum16{"Init", "Set", "Get"}."Set") -> ()  [unwired: 10 in, 7 out]
          }
        }
      }
    }
  }
